vi "Get Waveform Type.vi"(8 "error in (no error)":errorcluster, 11 "VISA resource name":refnum<visa-resource-name>) -> (0 "error out":errorcluster {"code" format="%.0x"}, 1 "2nd Waveform":i32, 2 "1st Waveform":i32, 3 "VISA resource name out":refnum<visa-resource-name>)   [LabVIEW 2013, in "Fluke 5XXX Series Multicalibrators.lvlib"]
doc: "This VI returns the waveform types for ac outputs. Waveform choices are SINE (sinewave), TRI (trianglewave), SQUARE (squarewave), TRUNCS (truncated sinewave), or NONE (waveform does not apply).\n\nNote:\n\nThis VI is available only for instrument models 5500A and 5520A."
uses:
  Fluke 5XXX Series Multicalibrators.lvlib
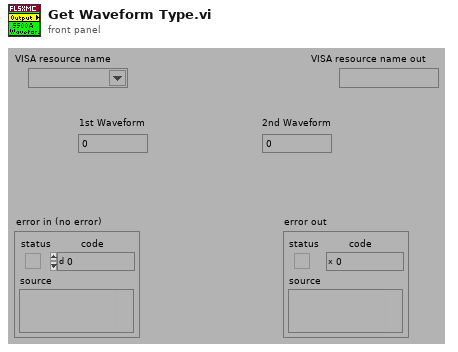
[diagram p1: front panel]
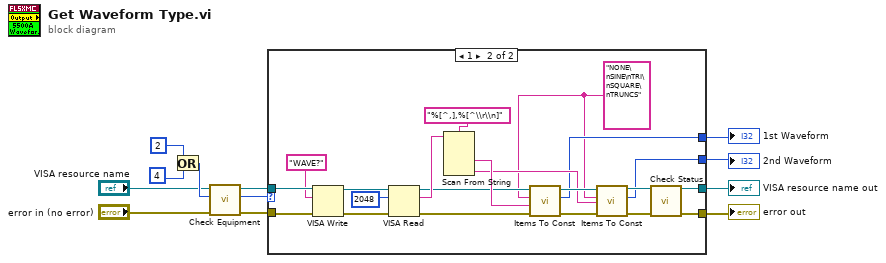
[diagram p0: block diagram]
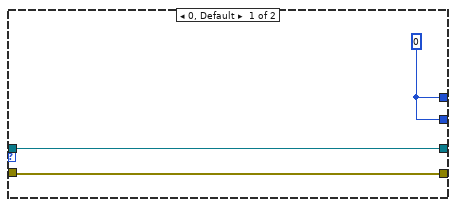
[diagram p2: hidden frame]
diagram:
  n1 = Or(x=2 ("Numeric"), y=4 ("Numeric")) -> (x .or. y?=w9:i32)
  n2 = call "Check Equipment.vi"("error in (no error)"="error in (no error)", "Bit Mask"=w9, "VISA resource name"="VISA resource name") -> ("error out"=w12:errorcluster, "Present?"=w11:u32, "VISA resource name out"=w10:refnum<visa-resource-name>)  [unwired: 6 in]
  n3 = case shown="1" w11 {
    tunnel: [w14 w19] -> w3
    tunnel: w12 -> [w15 w36]
    tunnel: w10 -> [w14 w35]
    tunnel: [w15 w24] -> w6
    tunnel: [w13 w18] -> w2
    tunnel: [w13 w17] -> w1
    frame 0, Default {
      w13 = u16 0 ("f")
    }
    frame 1 {
      w16 = "NONE\nSINE\nTRI\nSQUARE\nTRUNCS"
      n4 = VISA Write(VISA resource name=w35, write buffer="WAVE?", error in (no error)=w36) -> (VISA resource name out=w32:refnum<visa-resource-name>, error out=w31:errorcluster)  [unwired: 1 out]
      n5 = VISA Read(VISA resource name=w32, byte count=u32 2048 ("byte count (0)"), error in (no error)=w31) -> (VISA resource name out=w21:refnum<visa-resource-name>, read buffer=w29:string, error out=w22:errorcluster)  [unwired: 1 out]
      n6 = Scan From String(format string="%[^,],%[^\\r\\n]", input string=w29) -> (output 1=w26:string, output 2=w25:string)  [unwired: 4 in, 3 out]
      n7 = call "Items To Const.vi"("error in (no error)"=w22, "String Item"=w26, "Multi-Line String"=w16, "VISA resource name"=w21) -> ("error out"=w28:errorcluster, "Index"=w18:i32, "VISA resource name out"=w27:refnum<visa-resource-name>)  [unwired: 5 in]
      n8 = call "Items To Const.vi"("error in (no error)"=w28, "String Item"=w25, "Multi-Line String"=w16, "VISA resource name"=w27) -> ("error out"=w23:errorcluster, "Index"=w17:i32, "VISA resource name out"=w20:refnum<visa-resource-name>)  [unwired: 5 in]
      n9 = call "Check Status.vi"("VISA resource name"=w20, "error in (no error)"=w23) -> ("VISA resource name out"=w19:refnum<visa-resource-name>, "error out"=w24:errorcluster)  [unwired: 12 in]
    }
  }
  "1st Waveform" <- w2
  "2nd Waveform" <- w1
  "VISA resource name out" <- w3
  "error out" <- w6
